vi "Do.vi"(8 "error in (no error)":errorcluster, 10 "Actor in":refnum<class "Actor.lvclass">, 11 "User Event-Panel Resize Msg":refnum<class "User Event-Panel Resize Msg.lvclass">) -> (0 "error out":errorcluster, 2 "Actor out":refnum<class "Actor.lvclass">)   [LabVIEW 2021, in "Appearance Actor.lvlib" / "User Event-Panel Resize Msg.lvclass"]
doc: "This VI delivers the message to the actor by calling the appropriate method(s) on the actor."
uses:
  User Event-Panel Resize Msg.lvclass
  <vilib>/ActorFramework/Actor/Actor.lvclass
  User Event-Panel Resize Msg.lvclass/User Event-Panel Resize Msg.ctl
  Appearance Actor/Appearance Actor.lvclass
  C:/Program Files (x86)/National Instruments/LabVIEW 2021/vi.lib/ActorFramework/Actor/Actor.lvclass
  0a4dab9a-2fe3-4756-a0d9-1e1ce3f8f978.vi
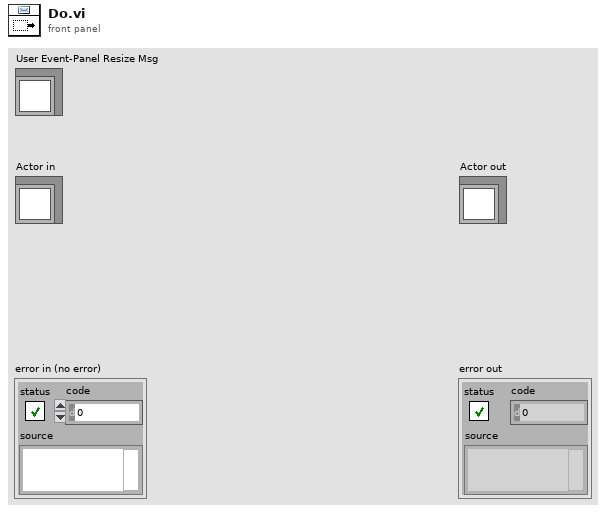
[diagram p1: front panel]
types:
  T1 = typedef "Appearance Actor.lvlib/Appearance Actor.lvclass/User Event-Panel Resize-Data--cluster.ctl" = cluster{"OldBnds":T2, "NewBnds":T2, "Act":T3, "PrevState":T4}
  T2 = typedef "LVRectTypeDef.ctl" = cluster{"Left":i16, "Top":i16, "Right":i16, "Bottom":i16}
  T3 = typedef "sizeaction.ctl" = enum32{"Minimized", "Maximized", "Resized"}
  T4 = typedef "panelstate.ctl" = enum32{"Standard", "Minimized", "Maximized"}
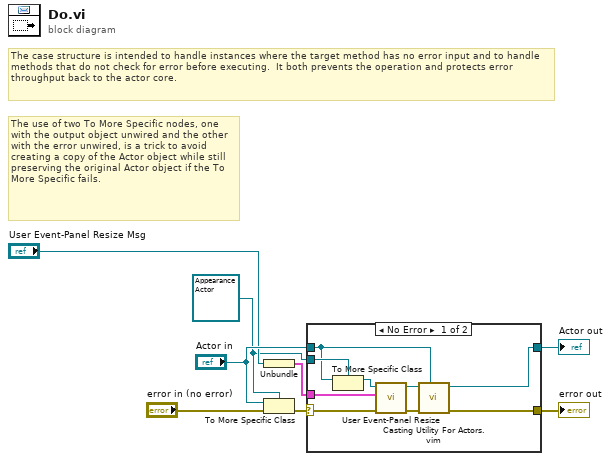
[diagram p0: block diagram]
diagram:
  w3 = refnum<class "Appearance Actor.lvclass"> refnum ("Actor in")
  # "The use of two To More Specific nodes, one with the output object unwired and the other with the error unwired, is a trick to avoid creating a copy of the Actor object while still preserving the original Actor object if the To More Specific fails."
  # "The case structure is intended to handle instances where the target method has no error input and to handle methods that do not check for error before executing.  It both prevents the operation and protects error throughput back to the actor core."
  n1 = Unbundle("User Event-Panel Resize Msg") -> (w1:T1)
  n2 = To More Specific Class(target class=w3, reference="Actor in", error in="error in (no error)") -> (error out=w2:errorcluster)  [unwired: 1 out]
  n3 = case shown="No Error" w2 {
    selector: w2 -> [w17 w19]
    tunnel: [w11 w19] -> w8
    tunnel: [w12 w18] -> w7
    tunnel: "Actor in" -> [w14 w18]
    tunnel: w3 -> [w15 _]
    tunnel: w1 -> [w9 _]
    frame No Error {
      n4 = To More Specific Class(target class=w15, reference=w14) -> (specific class reference=w16:refnum<class "Appearance Actor.lvclass">)  [unwired: 1 in, 1 out]
      n5 = call-dynamic "User Event-Panel Resize.vi"("Error In"=w17, "Panel Resize Data"=w9, "Appearance Actor in"=w16) -> ("Error Out"=w10:errorcluster, "Appearance Actor out"=w13:refnum<class "Appearance Actor.lvclass">)  [unwired: 7 in]
      n6 = call "Casting Utility For Actors.vim"("type"=w14, "error in (no error)"=w10, "Actor in"=w13) -> ("error out"=w11:errorcluster, "Actor out"=w12:refnum<class "Actor.lvclass">)  [unwired: 7 in]
    }
    frame Error {
      # "If type check fails, pass the original object out again."
    }
  }
  "error out" <- w8
  "Actor out" <- w7
